vi "Out_S1F14.vi"(7 "Host":bool, 8 "error in (no error)":errorcluster, 10 "S1F14":T1, 11 "S1 Message Class in":refnum<class "S1 Message Class.lvclass">) -> (0 "error out":errorcluster, 3 "S1 Message Class out":refnum<class "S1 Message Class.lvclass">)   [LabVIEW 2020, in "SECS Communication.lvlib" / "S1 Message Class.lvclass"]
uses:
  S1 Message Class.lvclass
  D:/Dropbox/SECS/SECS_GEM v1.1.0/Com/SECS Communication/SECS-II Class/SECS-II Class.lvclass
  S1F14.ctl
  SECS-II Class/Data Message_List.vi
  SECS-II Class/Data Message_Binary.vi
  SECS-II Class/Data Message_ASCII.vi
  SECS-II Class/SECS-II Class.lvclass
  D:/Dropbox/SECS/SECS_GEM v1.1.0/Com/SECS Communication/S1 Message Class/S1 Message Class.lvclass
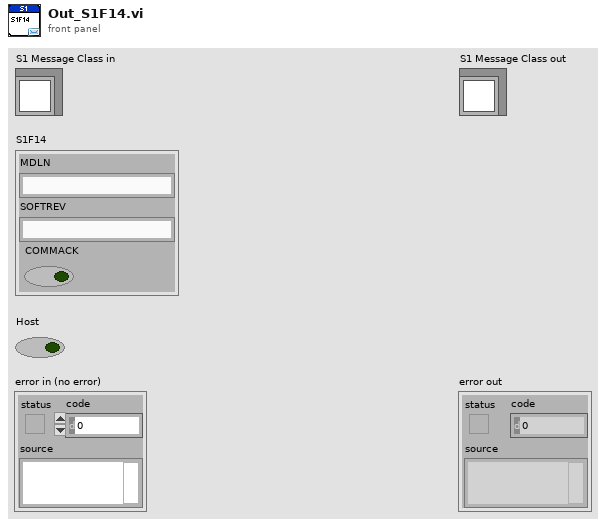
[diagram p1: front panel]
types:
  T1 = typedef "SECS Communication.lvlib/S1 Message Class.lvclass/S1F14.ctl" = cluster{"MDLN":string, "SOFTREV":string, "COMMACK":bool}
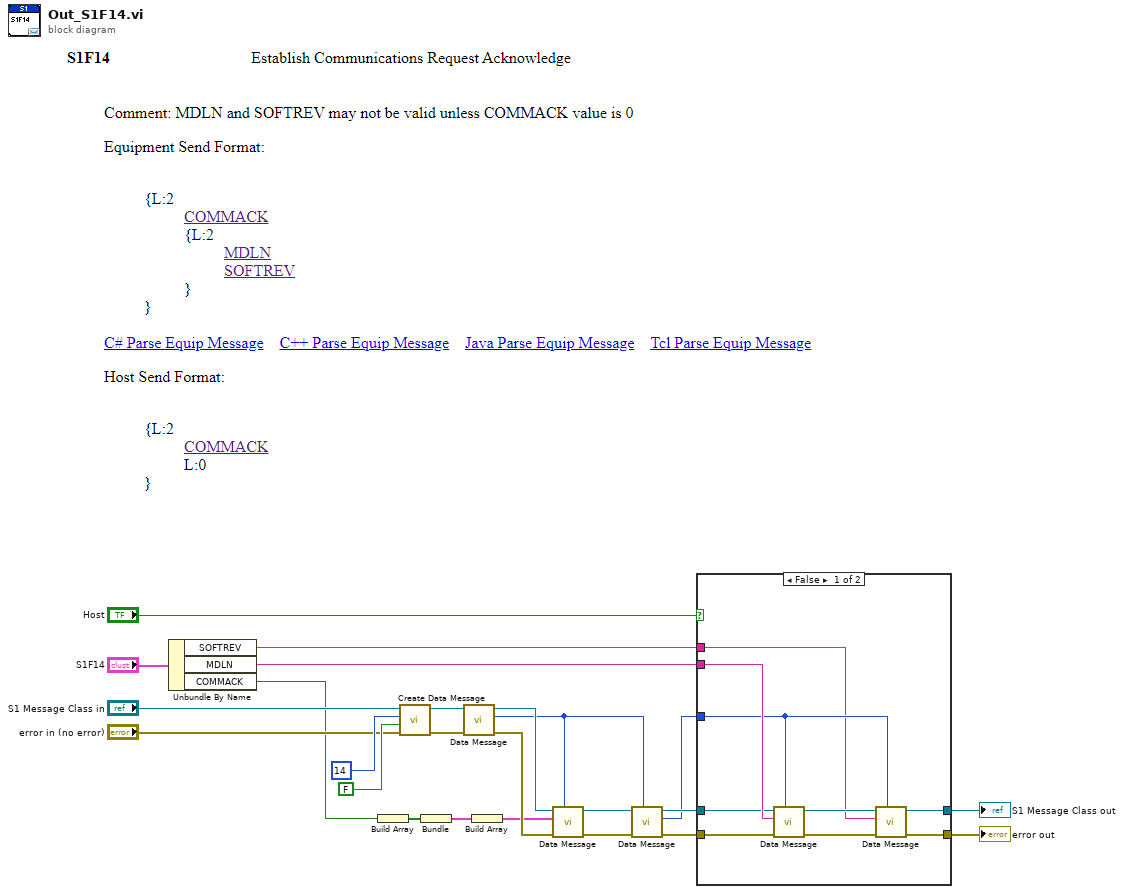
[diagram p0: block diagram]
diagram:
  n1 = Unbundle By Name("S1F14") -> ("SOFTREV"=w4:string, "MDLN"=w3:string, "COMMACK"=w2:bool)
  n2 = Build Array(w2) -> (w14:bool[])
  n3 = call "Create Data Message.vi"("error in (no error)"="error in (no error)", "W-Bit"=FALSE, "Function"=u8 14, "SECS-II Class in"="S1 Message Class in") -> ("error out"=w19:errorcluster, "SECS-II Class out"=w20:refnum<class "S1 Message Class.lvclass">)  [unwired: 6 in]
  n4 = Bundle(w14) -> (w13:cluster{bool[]})  [unwired: 1 in]
  n5 = call-poly "Data Message.vi"("error in"=w19, "SECS-II Class in"=w20) -> ("error out"=w16:errorcluster, "Index"=w9:i32, "SECS-II Class out"=w15:refnum<class "S1 Message Class.lvclass">)  [unwired: 7 in]
  n6 = Build Array(w13) -> (w12:cluster{bool[]}[])
  n7 = call-poly "Data Message.vi"("Parent Index"=w9, "error in"=w16, "Data Cluster"=w12, "SECS-II Class in"=w15) -> ("error out"=w11:errorcluster, "SECS-II Class out"=w10:refnum<class "S1 Message Class.lvclass">)  [unwired: 6 in]
  n8 = call-poly "Data Message.vi"("Parent Index"=w9, "error in"=w11, "SECS-II Class in"=w10) -> ("error out"=w8:errorcluster, "Index"=w6:i32, "SECS-II Class out"=w7:refnum<class "S1 Message Class.lvclass">)  [unwired: 6 in]
  n9 = case shown="False" "Host" {
    tunnel: w8 -> [w33 w35]
    tunnel: w3 -> [w32 _]
    tunnel: w6 -> [w29 _]
    tunnel: w4 -> [w28 _]
    tunnel: [w27 w35] -> w18
    tunnel: [w26 w34] -> w1
    tunnel: w7 -> [w25 w34]
    frame False {
      n10 = call-poly "Data Message.vi"("Parent Index"=w29, "error in"=w33, "Data"=w32, "SECS-II Class in"=w25) -> ("error out"=w30:errorcluster, "SECS-II Class out"=w31:refnum<class "S1 Message Class.lvclass">)  [unwired: 6 in]
      n11 = call-poly "Data Message.vi"("Parent Index"=w29, "error in"=w30, "Data"=w28, "SECS-II Class in"=w31) -> ("error out"=w27:errorcluster, "SECS-II Class out"=w26:refnum<class "S1 Message Class.lvclass">)  [unwired: 6 in]
    }
    frame True {
    }
  }
  "error out" <- w18
  "S1 Message Class out" <- w1
